vi "Read linear_kick_work_.vi"(8 "error in (no error)":errorcluster, 11 "Robot in":refnum<class "Robot.lvclass">) -> (0 "error out":errorcluster, 2 "linear_kick_work?":T1, 3 "Robot out":refnum<class "Robot.lvclass">)   [LabVIEW 2022 SP3, in "Robot.lvclass"]
uses:
  Robot.lvclass
  chip_kick.ctl
  Robot.lvclass/Robot.ctl
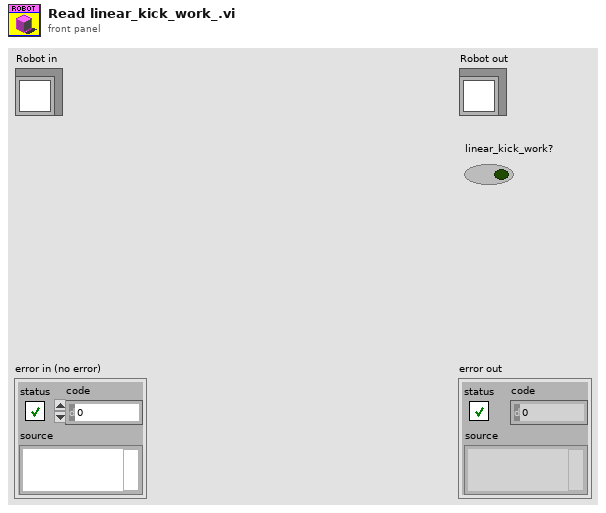
[diagram p1: front panel]
types:
  T1 = typedef "chip_kick.ctl" = bool
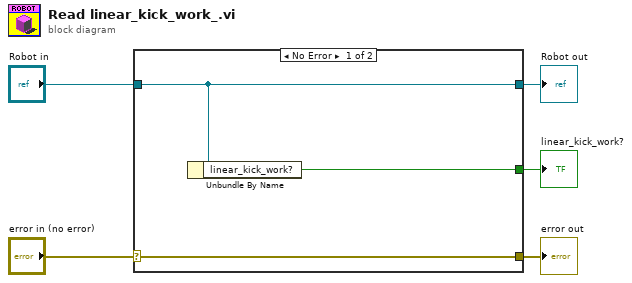
[diagram p0: block diagram]
diagram:
  n1 = case shown="No Error" "error in (no error)" {
    selector: "error in (no error)" -> [w8 w9]
    tunnel: [w8 w9] -> w4
    tunnel: [w7 w10] -> w2
    tunnel: "Robot in" -> [w7 w10]
    tunnel: [w6 _] -> w1
    frame No Error {
      n2 = Unbundle By Name(w7) -> ("linear_kick_work?"=w6:T1)
    }
    frame Error {
    }
  }
  "error out" <- w4
  "Robot out" <- w2
  "linear_kick_work?" <- w1
